vi "706 neustart.vi"(8 "error in (no error)":errorcluster) -> (0 "error out":errorcluster)   [LabVIEW 2014]
uses:
  <vilib>/CANopenLib/CANOPEN.llb/CANopen Interface Close.vi
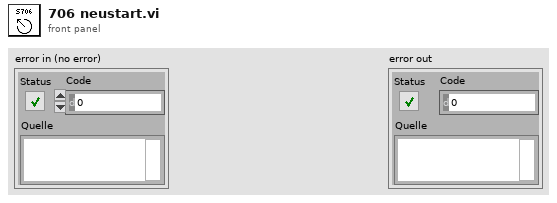
[diagram p1: front panel]
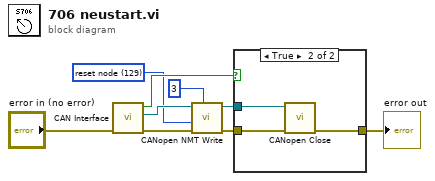
[diagram p0: block diagram]
diagram:
  w4 = u16 129 items=["start remote node"=1, "stop remote node"=2, "enter pre-operational"=128, "reset node"=129, "reset communication"=130] ("command")
  n1 = call "CAN Interface.vi"("error in (no error)"="error in (no error)") -> ("error out"=w5:errorcluster, "interface object out"=w6:refnum<k20>, "Interface schließen?"=w8:bool)  [unwired: 8 in]
  n2 = call <vilib>:"CANopen NMT Write.vi"("node-ID (0)"=u8 3, "error in (no error)"=w5, "command"=w4, "interface object in"=w6) -> ("error out"=w1:errorcluster, "interface object out"=w2:refnum<k20>)  [unwired: 6 in]
  n3 = case shown="True" w8 {
    tunnel: w1 -> [w10 w13]
    tunnel: w2 -> [_ w12]
    tunnel: [w10 w11] -> w7
    frame False {
    }
    frame True {
      n4 = call-poly <vilib>:"CANopen Close.vi"("error in (no error)"=w13, "interface object in"=w12) -> ("error out"=w11:errorcluster)  [unwired: 9 in]
    }
  }
  "error out" <- w7
